vi "Reinitialize Front Panel.vi"(8 "error in (no error)":errorcluster, 9 "error in":errorcluster, 10 "This VI":refnum<vi>, 11 "Tab Control In":refnum<vi>) -> (0 "error out":errorcluster)   [LabVIEW 2021]
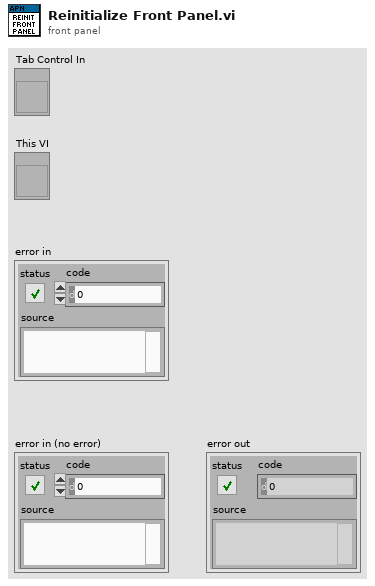
[diagram p1: front panel]
types:
  T1 = enum32{"Page Enabled", "Page Disabled", "Page Disabled & Grayed"}
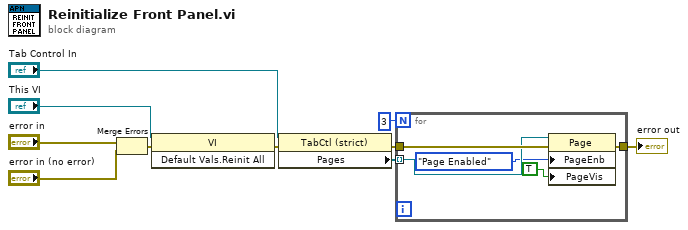
[diagram p0: block diagram]
diagram:
  n1 = Merge Errors("error in", "error in (no error)") -> (w9:errorcluster)
  n2 = invoke class="VI" method="Default Vals.Reinit All"(reference="This VI", error in=w9) -> (error out=w10:errorcluster)  [unwired: 1 in, 2 out]
  n3 = property on="Property Node" class="TabCtl (strict)"(reference="Tab Control In", error in=w10) -> (error out=w4:errorcluster, "Pages"=w6:refnum<vi>[])  [unwired: 1 out]
  n4 = for {
    N: 3 -> [_]
    tunnel: w4 -> [w15]
    tunnel: [w14] -> w5
    tunnel: w6 -> [w13] mode=indexing
    n5 = property class="Page"(reference=w13, error in=w15, "PageEnb"=T1."Page Enabled" ("Page Enabled State"), "PageVis"=TRUE ("Page Visible")) -> (error out=w14:errorcluster)  [unwired: 1 out]
  }
  "error out" <- w5
